vi "KelvinToCelcuis.vi"(11 "Кельвин":dbl) -> (3 "Цельсий":dbl)   [LabVIEW 2017]
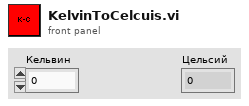
[diagram p1: front panel]
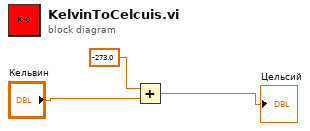
[diagram p0: block diagram]
diagram:
  n1 = Add(x=-273.0, y="Кельвин") -> (x+y=→"Цельсий":dbl)
